vi "Cobro.vi"(8 "error in (no error)":errorcluster, 10 "Numeric":dbl, 11 "Monedas in":refnum<class "Monedas.lvclass">) -> (0 "error out":errorcluster, 3 "Monedas out":refnum<class "Monedas.lvclass">)   [LabVIEW 2020, in "Monedas.lvlib" / "Monedas.lvclass"]
uses:
  Monedas.lvclass
  <vilib>/ActorFramework/Actor/Actor.lvclass
  UI Messages/Dinero Update Msg/Dinero Update Msg.lvclass
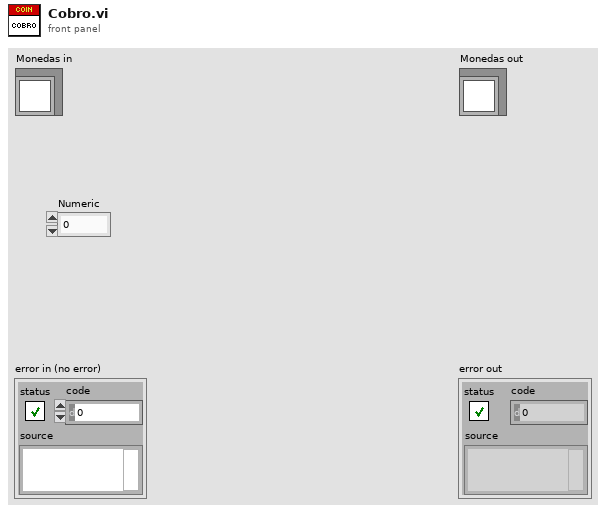
[diagram p1: front panel]
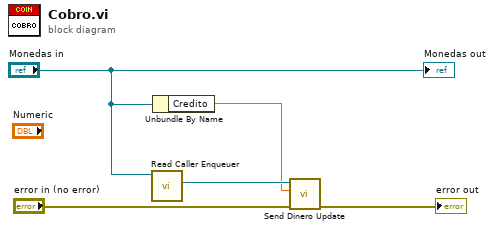
[diagram p0: block diagram]
diagram:
  n1 = call <vilib>:"Read Caller Enqueuer.vi"("Actor"="Monedas in") -> ("Caller Enqueuer"=w4:refnum<class "Message Enqueuer.lvclass">)  [unwired: 10 in]
  n2 = Unbundle By Name("Monedas in") -> ("Credito"=w3:dbl)
  n3 = call "Send Dinero Update.vi"("error in (no error)"="error in (no error)", "Dinero"=w3, "Message Enqueuer"=w4) -> ("error out"=→"error out":errorcluster)  [unwired: 7 in, 1 out]
  "Monedas out" <- "Monedas in"
